vi "SigProc_method pyProcess.vi"(5 "replace?(T)":bool=TRUE, 7 "func":T1(ring), 8 "error in (no error)":errorcluster, 10 "newScriptCode":string, 11 "dataParam":T2) -> (0 "error out":errorcluster, 2 "pyCode":string, 3 "newSigInfo":T3, 4 "showMsg":string[](array[string]))   [LabVIEW 2018, in "Sig2MS.lvclass"]
uses:
  Sig2MS.lvclass
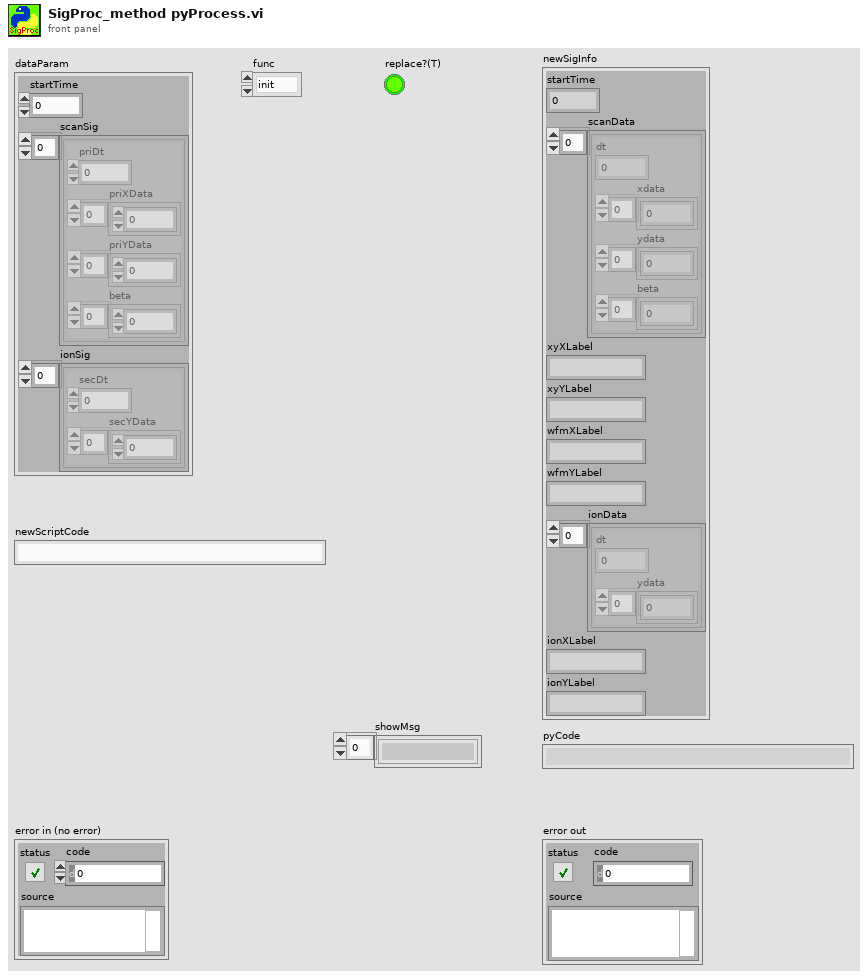
[diagram p1: front panel]
types:
  T1 = enum16{"init", "loadScript", "newScript", "runScript", "close"}
  T2 = cluster{"startTime":dbl, "scanSig":cluster{"priDt":dbl, "priXData":dbl[], "priYData":sgl[], "beta":dbl[]}[], "ionSig":cluster{"secDt":dbl, "secYData":sgl[]}[]}
  T3 = cluster{"startTime":dbl, "scanData":cluster{"dt":dbl, "xdata":dbl[], "ydata":sgl[], "beta":dbl[]}[], "xyXLabel":string, "xyYLabel":string, "wfmXLabel":string, "wfmYLabel":string, "ionData":cluster{"dt":dbl, "ydata":sgl[]}[], "ionXLabel":string, "ionYLabel":string}
  T4 = enum16{"open", "replace", "create", "open or create", "replace or create", "replace or create with confirmation"}
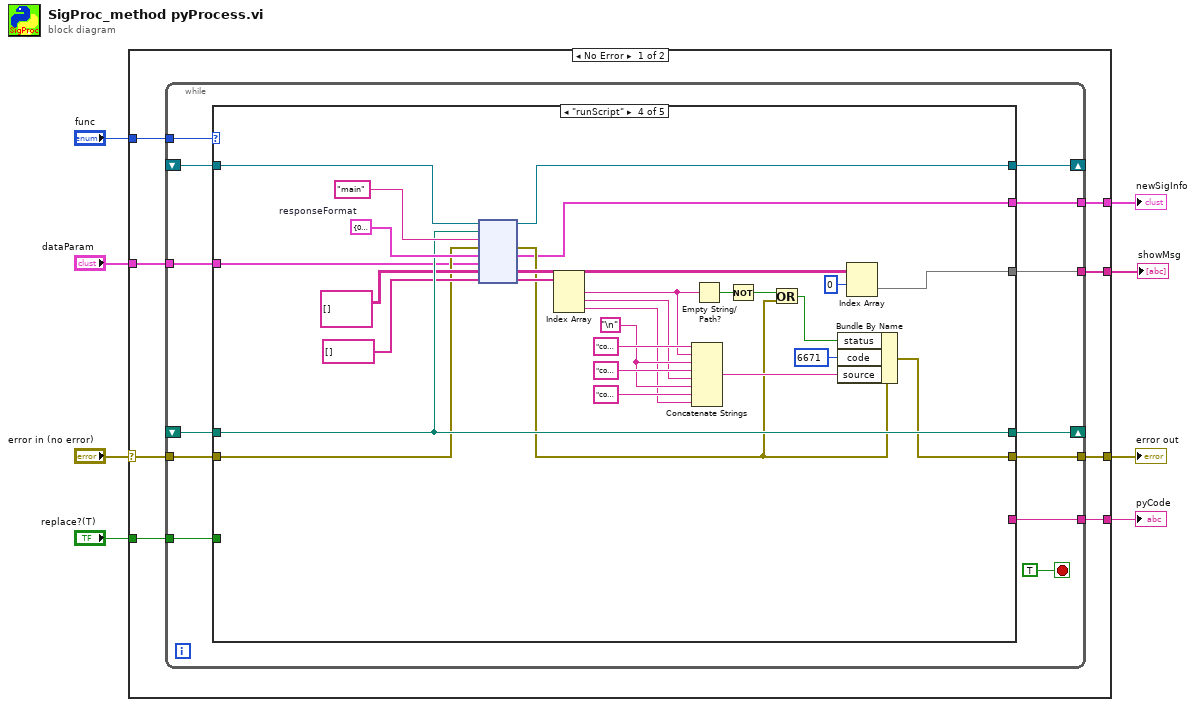
[diagram p0: block diagram]
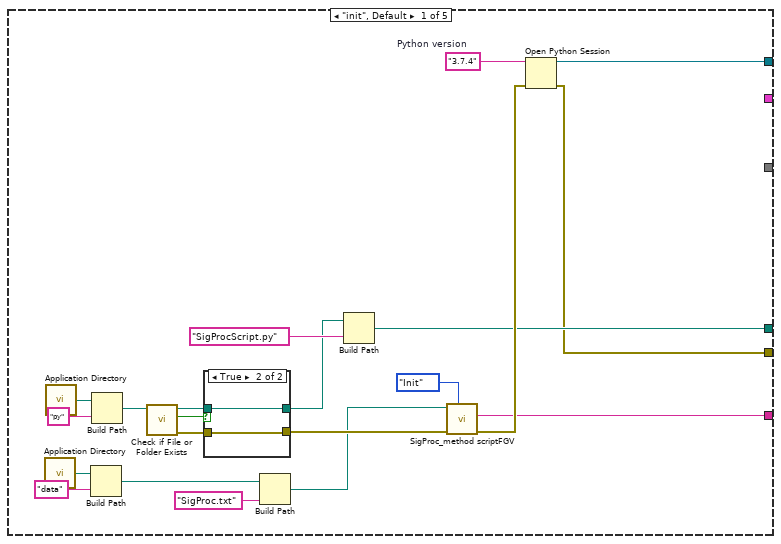
[diagram p2: hidden frame]
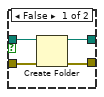
[diagram p3: hidden frame]
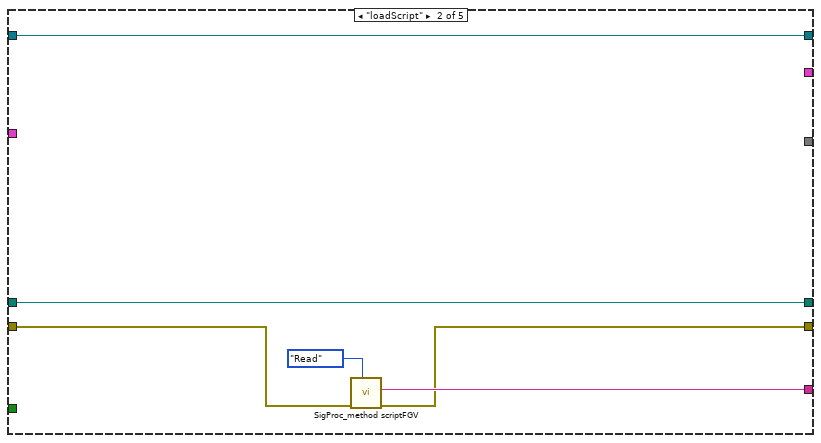
[diagram p4: hidden frame]
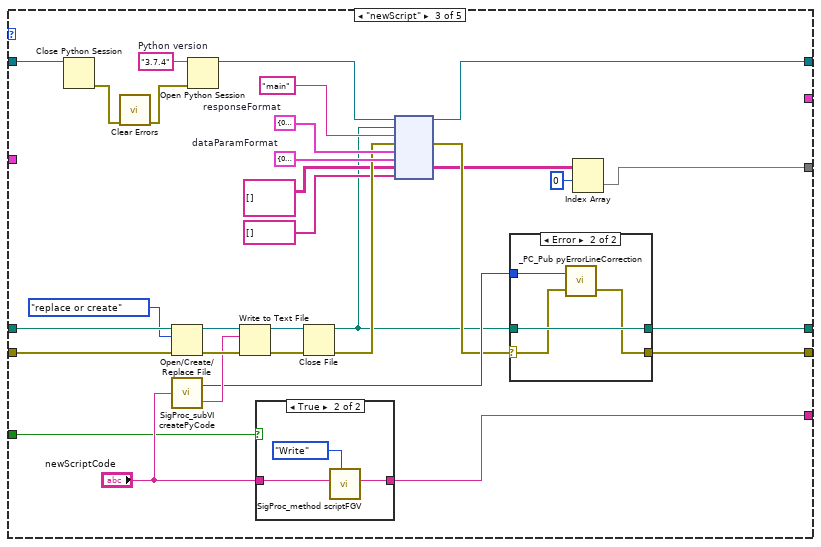
[diagram p5: hidden frame]
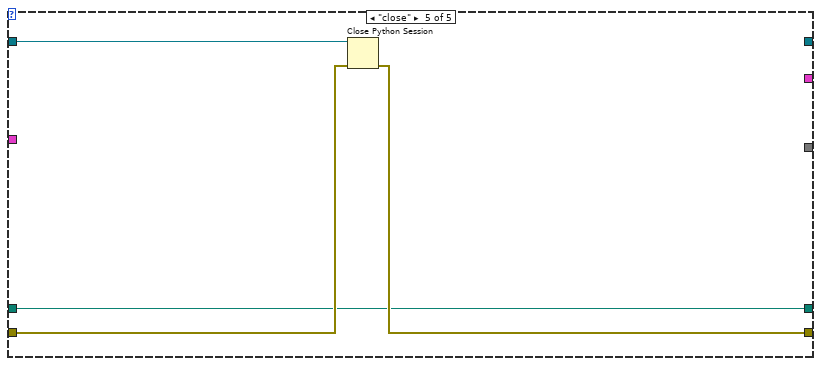
[diagram p8: hidden frame]
diagram:
  n1 = case shown="No Error" "error in (no error)" {
    selector: "error in (no error)" -> [w11 w136]
    tunnel: "func" -> [w16 _]
    tunnel: [w15 _] -> w7
    tunnel: [w14 _] -> w6
    tunnel: [w13 w136] -> w5
    tunnel: "dataParam" -> [w12 _]
    tunnel: "replace?(T)" -> [w10 _]
    tunnel: [w9 _] -> w1
    frame No Error {
      n2 = while {
        tunnel: w16 -> [w29]
        shift-right: [w28] -> _
        shift-left: _ -> [w27]
        shift-right: [w26] -> _
        shift-left: _ -> [w25]
        tunnel: [w23] -> w15
        tunnel: [w22] -> w14
        tunnel: w11 -> [w24]
        tunnel: [w20] -> w13
        tunnel: w12 -> [w19]
        tunnel: w10 -> [w18]
        tunnel: [w17] -> w9
        stop <- TRUE stop-if-true
        n3 = case shown="\"runScript\"" w29 {
          tunnel: [w49 w58 w81 w129 _] -> w28
          tunnel: w27 -> [_ w58 w78 w120 w135]
          tunnel: [w36 w59 w66 w106 w133] -> w20
          tunnel: [w37 w57 w67 w121 w132] -> w26
          tunnel: w25 -> [_ w57 w91 w121 w132]
          tunnel: w24 -> [_ w60 w90 w111 w134]
          tunnel: [w38 w61 w92 _ _] -> w23
          tunnel: [_ _ _ w104 _] -> w22
          tunnel: w19 -> [_ _ _ w105 _]
          tunnel: w18 -> [_ _ w79 _ _]
          tunnel: [_ _ w63 w115 _] -> w17
          frame "init", Default {
            w50 = "3.7.4"  # Python version
            n4 = call <vilib>:"Application Directory.vi"() -> ("Application Directory"=w32:path)
            n5 = call <vilib>:"Application Directory.vi"() -> ("Application Directory"=w47:path)
            n6 = Build Path(base path=w32, name or relative path="data") -> (appended path=w31:path)
            n7 = Build Path(base path=w47, name or relative path="py") -> (appended path=w34:path)
            n8 = call <vilib>:"Check if File or Folder Exists.vi"("path"=w34) -> ("error out"=w44:errorcluster, "file or folder exists?"=w46:bool, "dup path"=w45:path)  [unwired: 8 in]
            n9 = case shown="True" w46 {
              tunnel: w45 -> [w54 w56]
              tunnel: w44 -> [w53 w55]
              tunnel: [w52 w56] -> w42
              tunnel: [w51 w55] -> w40
              frame False {
                n10 = Create Folder(path (use dialog)=w54, error in=w53) -> (created path=w52:path, error out=w51:errorcluster)  [unwired: 1 in, 1 out]
              }
              frame True {
              }
            }
            n11 = Build Path(base path=w31, name or relative path="SigProc.txt") -> (appended path=w30:path)
            n12 = Build Path(base path=w42, name or relative path="SigProcScript.py") -> (appended path=w37:path)
            n13 = call "SigProc_method scriptFGV.vi"("Function"=enum16{"Read", "Write", "Init"}."Init", "error in"=w40, "dup path"=w30) -> ("error out"=w39:errorcluster, "Script out"=w38:string)  [unwired: 5 in]
            n14 = Open Python Session(python version=w50, 3:w39) -> (session out=w49:refnum<k35>, error out=w36:errorcluster)  [unwired: 1 in]
          }
          frame "loadScript" {
            n15 = call "SigProc_method scriptFGV.vi"("Function"=enum16{"Read", "Write", "Init"}."Read", "error in"=w60) -> ("error out"=w59:errorcluster, "Script out"=w61:string)  [unwired: 6 in]
          }
          frame "newScript" {
            w75 = "3.7.4"  # Python version
            w83 = T3 {"startTime"=0.0, "scanData"=[], "xyXLabel"="", "xyYLabel"="", "wfmXLabel"="", "wfmYLabel"="", "ionData"=[], "ionXLabel"="", "ionYLabel"=""}  # responseFormat
            w84 = T2 {"startTime"=0.0, "scanSig"=[], "ionSig"=[]}  # dataParamFormat
            n16 = Close Python Session(session in=w78) -> (11:w77:errorcluster)  [unwired: 1 in]
            n17 = call <vilib>:"Clear Errors.vi"("error in (no error)"=w77) -> ("error out"=w76:errorcluster)  [unwired: 5 in, 1 out]
            n18 = Open/Create/Replace File(file path (use dialog)=w91, error in=w90, operation (0:open)=T4."replace or create") -> (refnum out=w89:refnum<file>, error out=w88:errorcluster)  [unwired: 3 in, 1 out]
            n19 = call "SigProc_subVI createPyCode.vi"("newScriptCode"="newScriptCode") -> ("scriptStartIdx"=w70:i32, "pyCode"=w87:string)
            n20 = Open Python Session(python version=w75, 3:w76) -> (session out=w74:refnum<k35>)  [unwired: 1 in, 1 out]
            n21 = Write to Text File(file (use dialog)=w89, text=w87, error in=w88) -> (refnum out=w86:refnum<file>, error out=w85:errorcluster)  [unwired: 1 in, 1 out]
            n22 = case shown="True" w79 {
              tunnel: "newScriptCode" -> [w100 w102]
              tunnel: [w100 w101] -> w92
              frame False {
              }
              frame True {
                n23 = call "SigProc_method scriptFGV.vi"("Function"=enum16{"Read", "Write", "Init"}."Write", "Script in"=w102) -> ("Script out"=w101:string)  [unwired: 6 in, 1 out]
              }
            }
            n24 = Close File(refnum=w86, error in=w85) -> (path=w68:path, error out=w73:errorcluster)
            n25 = node(w74, w68, "main" ("function name"), w73, w83, w84, string[][] [], string[] []) -> (w81:refnum<k35>, w69:errorcluster, w64:string[][])  [unwired: 3 in, 2 out]
            n26 = case shown="Error" w69 {
              selector: w69 -> [w94 w97]
              tunnel: [w95 w99] -> w67
              tunnel: w68 -> [w95 w99]
              tunnel: [w94 w96] -> w66
              tunnel: w70 -> [_ w98]
              frame No Error {
              }
              frame Error {
                n27 = call "_PC_Pub pyErrorLineCorrection.vi"("error in (no error)"=w97, "scriptStartIdx"=w98) -> ("error out"=w96:errorcluster)  [unwired: 1 in]
              }
            }
            n28 = Index Array(array=w64, index (row)=0) -> (element=w63:string[])  [unwired: 1 in]
          }
          frame "runScript" {
            w126 = "\n"
            w131 = T3 {"startTime"=0.0, "scanData"=[], "xyXLabel"="", "xyYLabel"="", "wfmXLabel"="", "wfmYLabel"="", "ionData"=[], "ionXLabel"="", "ionYLabel"=""}  # responseFormat
            n29 = node(w120, w121, "main" ("function name"), w111, w131, w105, string[][] [], string[] []) -> (w129:refnum<k35>, w107:errorcluster, w104:T3, w116:string[][], w118:string[])  [unwired: 1 in, 2 out]
            n30 = Index Array(array=w118) -> (element #1=w122:string, element #2=w124:string, element #3=w123:string)  [unwired: 3 in]
            n31 = Concatenate Strings("codeError source : ", w122, w126, "codeError message : ", w124, w126, "codeError line : ", w123) -> (w108:string)
            n32 = Empty String/Path?(string/path=w122) -> (empty?=w112:bool)
            n33 = Not(x=w112) -> (.not. x?=w113:bool)
            n34 = Or(x=w113, y=w107) -> (x .or. y?=w110:bool)
            n35 = Bundle By Name(cluster=w107, "status"=w110, "code"=6671, "source"=w108) -> (w106:errorcluster)
            n36 = Index Array(array=w116, index (row)=0) -> (element=w115:string[])  [unwired: 1 in]
          }
          frame "close" {
            n37 = Close Python Session(session in=w135, error in=w134) -> (11:w133:errorcluster)
          }
        }
      }
    }
    frame Error {
    }
  }
  "error out" <- w5
  "pyCode" <- w7
  "newSigInfo" <- w6
  "showMsg" <- w1
